vi "DelayGeneratorController.vi"() -> ()   [LabVIEW 2009, in "DelayGenerator.lvlib"]
uses:
  DelayGenerator.lvlib
  Controls/DelayGeneratorState.ctl
  Aerotech/Controls/AerotechTarget.ctl
  Controls/DelayGeneratorCommand.ctl
panel:
  out "Target":T1
  out "State":T2
  in  "PROCESS":string="DELAYGENERATOR"
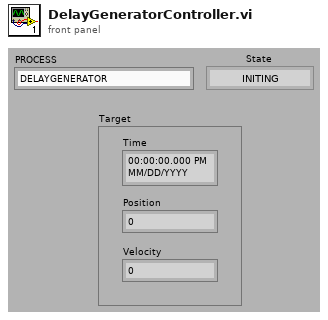
[diagram p1: front panel]
types:
  T1 = typedef "AerotechTarget.ctl" = cluster{"Time":timestamp, "Position":dbl, "Velocity":dbl}
  T2 = typedef "DelayGeneratorState.ctl" = enum16{"INITING", "IDLING", "TRACKING", "STOPPING"}
  T3 = typedef "DelayGeneratorCommand.ctl" = enum16{"IDLE", "TRACK", "QUIT"}
  T4 = typedef "DelayGeneratorSynchro.ctl" = cluster{"Command":refnum<queue>, "State":refnum<notifier>, "Offset":refnum<notifier>, "AerotechTarget":refnum<notifier>}
  T5 = typedef "DelayTarget.ctl" = cluster{"Time":timestamp, "Position":dbl[unit], "Velocity":dbl[unit]}
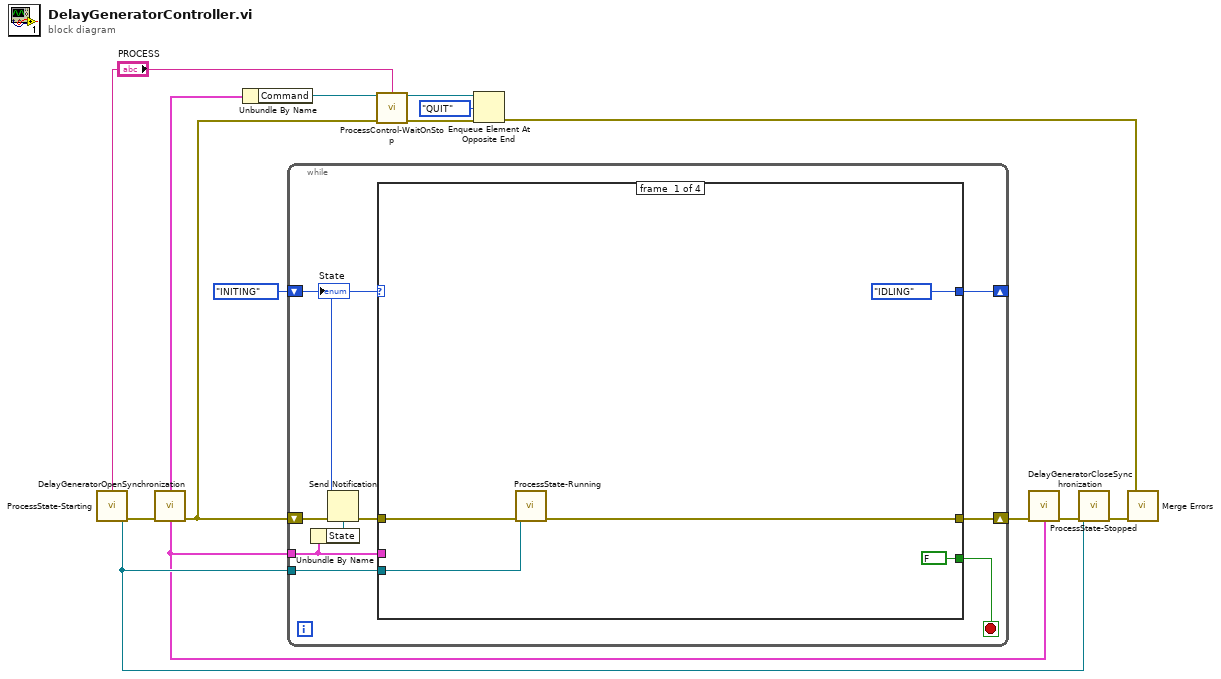
[diagram p0: block diagram]
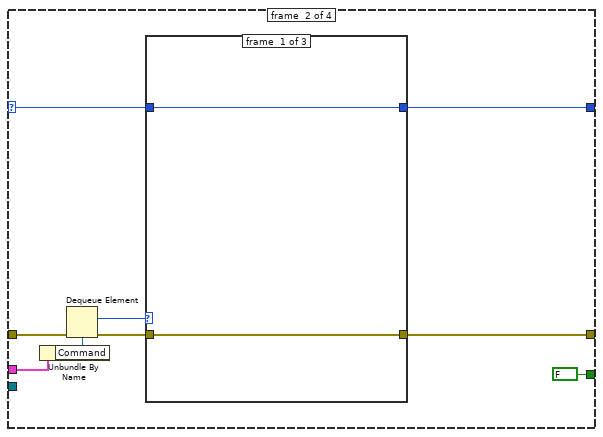
[diagram p2: hidden frame]
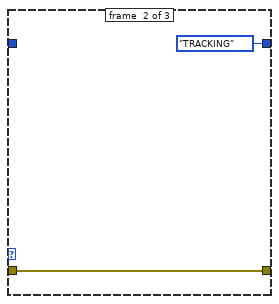
[diagram p3: hidden frame]
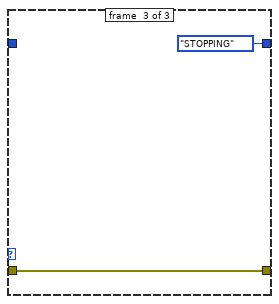
[diagram p4: hidden frame]
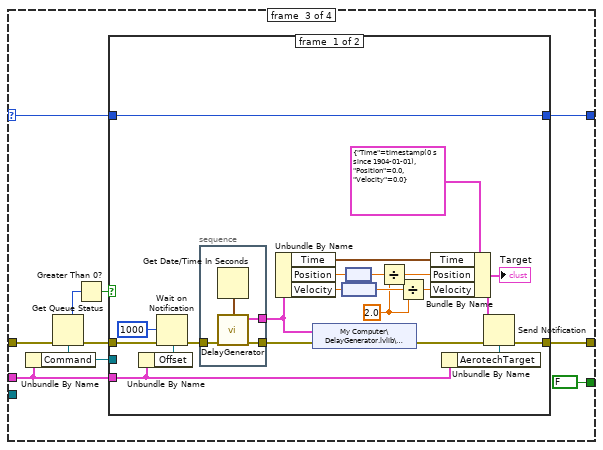
[diagram p5: hidden frame]
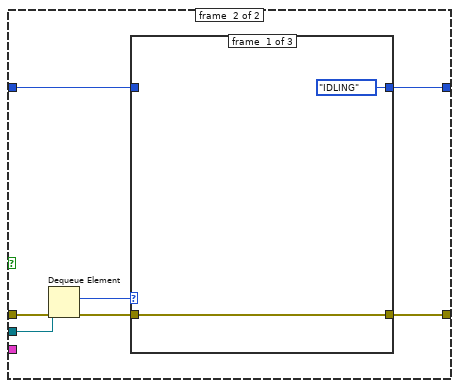
[diagram p6: hidden frame]
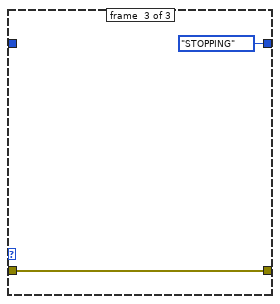
[diagram p8: hidden frame]
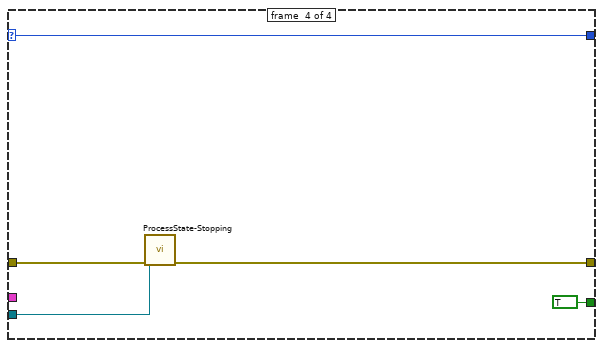
[diagram p9: hidden frame]
diagram:
  n1 = call "ProcessState-Starting.vi"("PROCESS"="PROCESS") -> ("ProcessStateNotifier"=w4:refnum<notifier>, "error in (no error)"=w13:errorcluster)  [unwired: 7 in]
  n2 = call "DelayGeneratorOpenSynchronization.vi"("error in (no error)"=w13) -> ("Synchro"=w1:T4, "error out"=w12:errorcluster)  [unwired: 7 in]
  n3 = Unbundle By Name(w1) -> ("Command"=w10:refnum<queue>)
  n4 = while {
    shift-right: [w15] -> w3
    shift-left: w12 -> [w19]
    shift-right: [w21] -> _
    shift-left: DelayGeneratorState."INITING" ("DelayGeneratorState") -> [w17]
    tunnel: w1 -> [w20]
    tunnel: w4 -> [w14]
    stop <- w22 stop-if-true
    n5 = Unbundle By Name(w20) -> ("State"=w18:refnum<notifier>)
    n6 = Send Notification(notification=w17, notifier=w18, error in (no error)=w19) -> (error out=w16:errorcluster)  [unwired: 1 out]
    n7 = case shown="\"TRACKING\"" w17 {
      selector: w17 -> [_ w31 w49 w94]
      tunnel: w16 -> [w26 w35 w52 w93]
      tunnel: w20 -> [_ w36 w46 _]
      tunnel: [FALSE FALSE FALSE TRUE] -> w22
      tunnel: [DelayGeneratorState."IDLING" ("DelayGeneratorState") w30 w44 w94] -> w21
      tunnel: [w25 w28 w43 w92] -> w15
      tunnel: w14 -> [w24 _ _ w91]
      frame #0 {
        n8 = call "ProcessState-Running.vi"("ProcessStateNotifier in"=w24, "error in (no error)"=w26) -> ("error out"=w25:errorcluster)  [unwired: 6 in, 1 out]
      }
      frame #1 {
        n9 = Unbundle By Name(w36) -> ("Command"=w34:refnum<queue>)
        n10 = Dequeue Element(queue=w34, error in (no error)=w35) -> (element=w33:T3, error out=w32:errorcluster)  [unwired: 1 in, 2 out]
        n11 = case shown="\"TRACK\"" w33 {
          tunnel: w32 -> [w38 w39 w42]
          tunnel: [w38 w39 w42] -> w28
          tunnel: w31 -> [w37 _ _]
          tunnel: [w37 DelayGeneratorState."TRACKING" ("DelayGeneratorState") DelayGeneratorState."STOPPING" ("DelayGeneratorState")] -> w30
          frame #0 {
          }
          frame #1 {
          }
          frame #2 {
          }
        }
      }
      frame #2 {
        n12 = Unbundle By Name(w46) -> ("Command"=w45:refnum<queue>)
        n13 = Get Queue Status(queue=w45, error in (no error)=w52) -> (error out=w48:errorcluster, # elements in queue=w51:i32)  [unwired: 1 in, 6 out]
        n14 = Greater Than 0?(x=w51) -> (x > 0?=w47:bool)
        n15 = case shown="False" w47 {
          tunnel: w49 -> [w61 w81]
          tunnel: w48 -> [w73 w84]
          tunnel: w46 -> [w69 _]
          tunnel: [w68 w79] -> w43
          tunnel: w45 -> [_ w83]
          tunnel: [w61 w80] -> w44
          frame #0 {
            w56 = 2.0 ("y")
            n16 = Unbundle By Name(w69) -> ("Offset"=w72:refnum<notifier>)
            n17 = Wait on Notification(notifier=w72, timeout in ms (-1)=1000, error in (no error)=w73) -> (error out=w70:errorcluster)  [unwired: 1 in, 3 out]
            n18 = stacked-sequence {
              tunnel: w70 -> [w77]
              tunnel: [w75] -> w55
              tunnel: [w74] -> w53
              frame #0 {
                n19 = Get Date/Time In Seconds() -> (seconds since 1Jan1904=w76:timestamp)
                n20 = call "DelayGenerator.vi"("error in (no error)"=w77, "Time Stamp"=w76) -> ("error out"=w75:errorcluster, "DelayTarget"=w74:T5)  [unwired: 8 in]
              }
            }
            n21 = Unbundle By Name(w53) -> ("Time"=w65:timestamp, "Position"=w63:dbl[unit], "Velocity"=w62:dbl[unit])
            n22 = shared-variable "My Computer\\DelayGenerator.lvlib\\DelayTarget"(w53, error in=w55) -> (error out=w54:errorcluster)
            n23 = node(w62) -> (w59:dbl)
            n24 = node(w63) -> (w58:dbl)
            n25 = Divide(x=w58, y=w56) -> (x/y=w60:dbl)
            n26 = Divide(x=w59, y=w56) -> (x/y=w57:dbl)
            n27 = Bundle By Name(cluster=T1 {"Time"=timestamp(0 s since 1904-01-01), "Position"=0.0, "Velocity"=0.0} ("notification"), "Time"=w65, "Position"=w60, "Velocity"=w57) -> (w64:T1)
            "Target" <- w64
            n28 = Unbundle By Name(w69) -> ("AerotechTarget"=w67:refnum<notifier>)
            n29 = Send Notification(notification=w64, notifier=w67, error in (no error)=w54) -> (error out=w68:errorcluster)  [unwired: 1 out]
          }
          frame #1 {
            n30 = Dequeue Element(queue=w83, error in (no error)=w84) -> (element=w82:T3, error out=w78:errorcluster)  [unwired: 1 in, 2 out]
            n31 = case shown="\"TRACK\"" w82 {
              tunnel: w81 -> [_ w88 _]
              tunnel: [DelayGeneratorState."IDLING" ("DelayGeneratorState") w88 DelayGeneratorState."STOPPING" ("DelayGeneratorState")] -> w80
              tunnel: [w85 w87 w89] -> w79
              tunnel: w78 -> [w85 w87 w89]
              frame #0 {
              }
              frame #1 {
              }
              frame #2 {
              }
            }
          }
        }
      }
      frame #3 {
        n32 = call "ProcessState-Stopping.vi"("ProcessStateNotifier in"=w91, "error in (no error)"=w93) -> ("error out"=w92:errorcluster)  [unwired: 6 in, 1 out]
      }
    }
    "State" <- w17
  }
  n33 = call "ProcessControl-WaitOnStop.vi"("PROCESS"="PROCESS", "error out"=w12) -> ("error in"=w11:errorcluster)  [unwired: 7 in]
  n34 = Enqueue Element At Opposite End(queue=w10, element=DelayGeneratorCommand."QUIT", error in (no error)=w11) -> (error out=w7:errorcluster)  [unwired: 1 in, 2 out]
  n35 = call "DelayGeneratorCloseSynchronization.vi"("Synchro"=w1, "error in (no error)"=w3) -> ("error out"=w2:errorcluster)  [unwired: 7 in]
  n36 = call "ProcessState-Stopped.vi"("ProcessStateNotifier in"=w4, "error in (no error)"=w2) -> ("error out"=w5:errorcluster)  [unwired: 7 in]
  n37 = call <vilib>:"Merge Errors.vi"("error in 3 (no error)"=w5, "error in 1 (no error)"=w7) -> ()  [unwired: 5 in, 1 out]
